vi "1.basic.vi"() -> ()   [LabVIEW 2018]
panel:
  out "Y":dbl
  in  "X":dbl
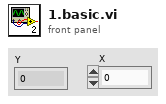
[diagram p1: front panel]
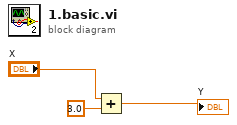
[diagram p0: block diagram]
diagram:
  n1 = Add(x="X", y=3.0) -> (x+y=→"Y":dbl)
